vi "STS_Cal_PDL.vi"(8 "错误输入（无错误）":errorcluster, 10 "ilData":sgl[][](array[numeric]), 11 ".NET引用句柄输入":refnum<k24>) -> (0 "error out":errorcluster, 3 "引用输出":refnum<k24>, 4 "minIL":sgl[](array[numeric]), 5 "il":sgl[](array[numeric]), 6 "maxIL":sgl[](array[numeric]), 7 "pdl":sgl[](array[numeric]))   [LabVIEW 2017]
doc: "Process ranges merge"
uses:
  D:/test/PDLSTS/LV_PDL LvVer17.0/LV_PDL_x64/DLL/STSProcess.dll
  DLL/STSProcess.dll
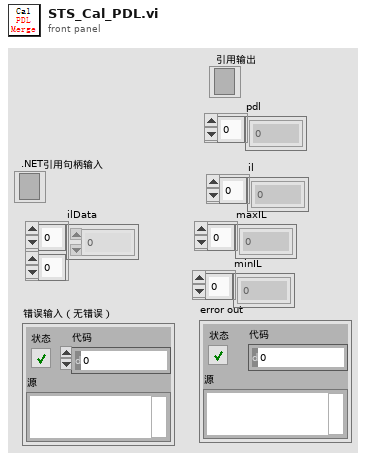
[diagram p1: front panel]
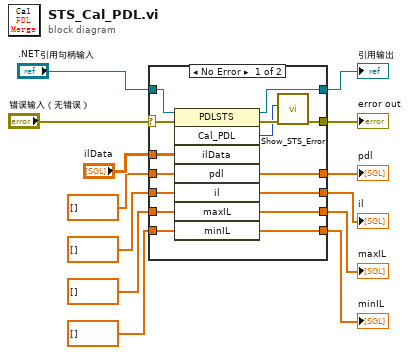
[diagram p0: block diagram]
diagram:
  n1 = case shown="No Error" "错误输入（无错误）" {
    selector: "错误输入（无错误）" -> [w27 w34]
    tunnel: ".NET引用句柄输入" -> [w28 w33]
    tunnel: [w24 w34] -> w11
    tunnel: [w23 w33] -> w10
    tunnel: "ilData" -> [w14 _]
    tunnel: [w22 w32] -> w8
    tunnel: [w21 w31] -> w7
    tunnel: [w20 w29] -> w6
    tunnel: [w19 w30] -> w5
    tunnel: sgl[] [] ("minIL") -> [w18 w29]
    tunnel: sgl[] [] ("maxIL") -> [w17 w30]
    tunnel: sgl[] [] ("il") -> [w16 w31]
    tunnel: sgl[] [] ("pdl") -> [w15 w32]
    frame No Error {
      n2 = invoke class="PDLSTS" method="Cal_PDL"(reference=w28, error in=w27, "ilData"=w14, "pdl"=w15, "il"=w16, "maxIL"=w17, "minIL"=w18) -> (reference out=w23:refnum<k24>, error out=w26:errorcluster, "Cal_PDL"=w25:i32, "pdl"=w22:sgl[], "il"=w21:sgl[], "maxIL"=w20:sgl[], "minIL"=w19:sgl[])  [unwired: 1 in, 1 out]
      n3 = call "Show_STS_Error.vi"("error in (no error)"=w26, "Error"=w25) -> ("error out"=w24:errorcluster)  [unwired: 9 in]
    }
    frame Error {
    }
  }
  "error out" <- w11
  "引用输出" <- w10
  "pdl" <- w8
  "il" <- w7
  "maxIL" <- w6
  "minIL" <- w5
